vi "DraftOCU.vi"() -> ()   [LabVIEW 2013]
doc: "Inputs from the control panel to the MDF \nOutputs an object\nWhen a button is pressed, creates and MDF object (based on information typed in by hand on the control panel) and adds it to a Q\nLimitations:????\nCreators: Bocamazo and Coleman\nDate:P 11/8/2013"
uses:
  RIO-OCU_Comm/NetworkStreams/Writer/NetworkStreamWriter.lvclass
  cRIO_Code/Logic/Classes/Missions/GenericMission/GenericMission.lvclass
  RIO-OCU_Comm/ToRIO.ctl
  Location of Think.ctl
  cRIO_Code/Data/TypeDefs/UTM Location.ctl
  cRIO_Code/Data/TypeDefs/MissionTypeControl.ctl
panel:
  in  "stop":bool
  in  "Mission Type":T1
  in  "Points of Interest":T2[](array[typedef]) {"North" format="%#_10f"; "East" format="%#_8f"}
  in  "Tolerance (m)":dbl
  in  "Duration (s)":dbl=-1.0
  in  "Timeout (s)":dbl=-1.0
  in  "OK Button":bool
  in  "Error In":errorcluster
  in  "stop 2":bool
  out "Connected?":bool
  in  "Location of THINK":T3="127.0.0.1"
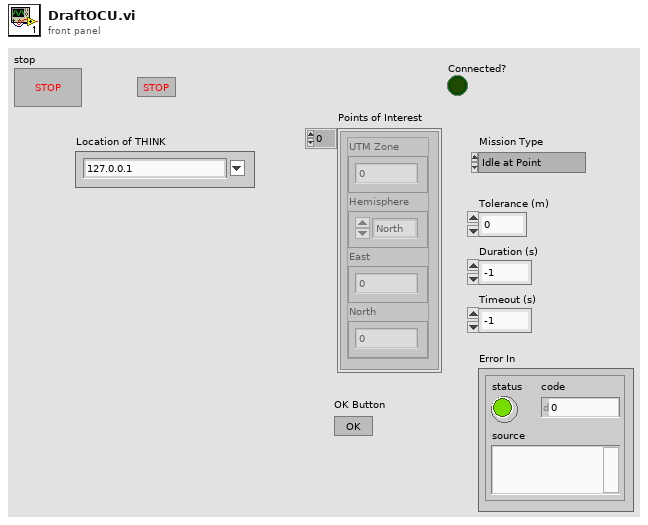
[diagram p1: front panel]
types:
  T1 = typedef "MissionTypeControl.ctl" = enum16{"Idle at Point", "Drive to Waypoint", "Round Buoy to Port", "Round Buoy to Starboard", "Pass Between Buoys", "Station Keeping"}
  T2 = typedef "UTM Location.ctl" = cluster{"UTM Zone":dbl, "Hemisphere":enum16{"North", "South"}, "East":dbl, "North":dbl}
  T3 = typedef "Location of Think.ctl" = string
  T4 = typedef "ToRIO.ctl" = cluster{"Mission":refnum<class "GenericMission.lvclass">}
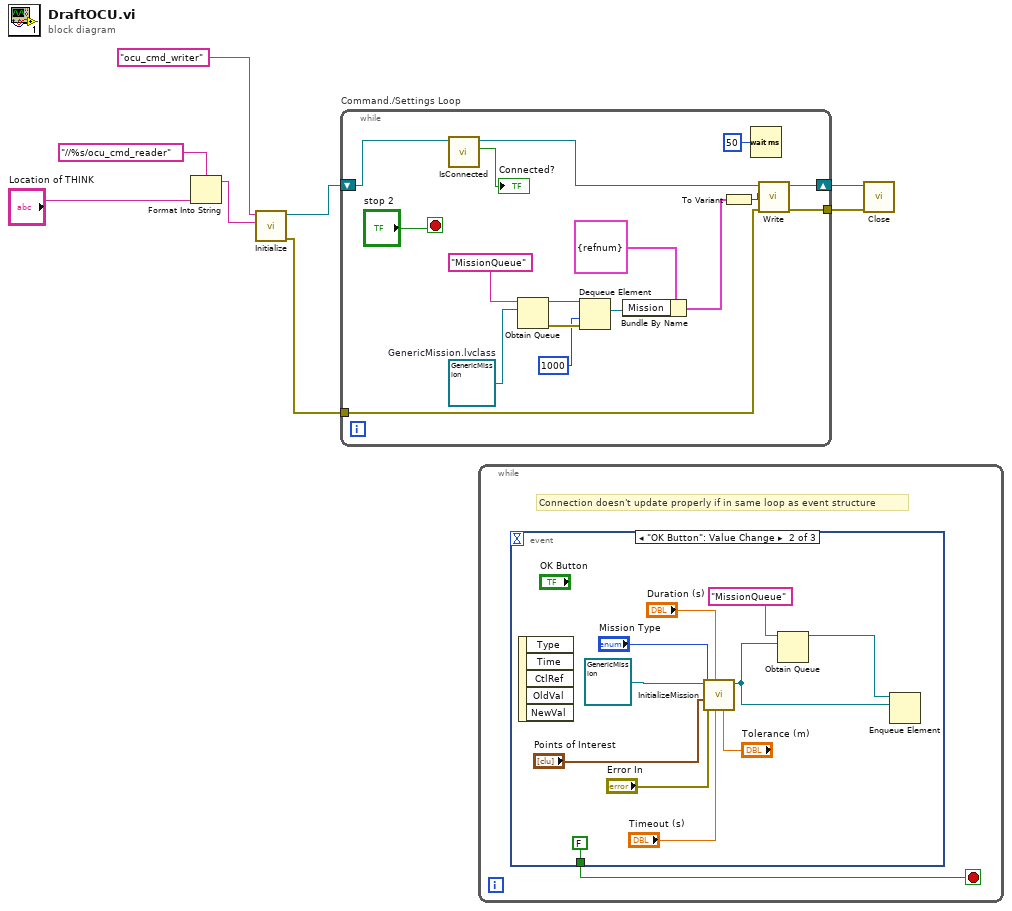
[diagram p0: block diagram]
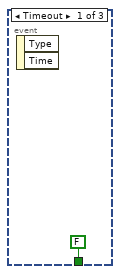
[diagram p2: hidden frame]
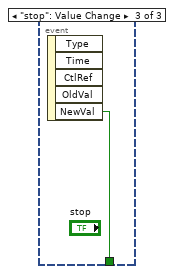
[diagram p3: hidden frame]
diagram:
  n1 = Format Into String(format string="//%s/ocu_cmd_reader", "Location of THINK") -> (resulting string=w7:string)  [unwired: 2 in, 1 out]
  n2 = call "Initialize.vi"("reader url"=w7, "writer name"="ocu_cmd_writer") -> ("error out"=w1:errorcluster, "NetworkStreamWriter out"=w2:refnum<class "NetworkStreamWriter.lvclass">)  [unwired: 8 in]
  n3 = while "Command./Settings Loop" {
    tunnel: [w16] -> w3
    shift-right: [w17] -> w4
    shift-left: w2 -> [w13]
    tunnel: w1 -> [w14]
    stop <- "stop 2" stop-if-true
    w18 = refnum<class "GenericMission.lvclass"> refnum  # GenericMission.lvclass
    n4 = call "IsConnected.vi"("NetworkStreamWriter in"=w13) -> ("Connected?"=→"Connected?":bool, "NetworkStreamWriter out"=w12:refnum<class "NetworkStreamWriter.lvclass">)  [unwired: 8 in, 1 out]
    n5 = Obtain Queue(name (unnamed)="MissionQueue", element data type=w18) -> (queue out=w24:refnum<queue>, error out=w23:errorcluster)  [unwired: 3 in, 1 out]
    n6 = Dequeue Element(queue=w24, timeout in ms (-1)=1000, error in (no error)=w23) -> (element=w22:refnum<class "GenericMission.lvclass">)  [unwired: 3 out]
    n7 = Bundle By Name(cluster=T4 {"Mission"=refnum} ("To RIO"), "Mission"=w22) -> (w19:T4)
    n8 = To Variant(anything=w19) -> (Variant=w20:variant)
    n9 = Wait (ms)(milliseconds to wait=u32 50) -> ()  [unwired: 1 out]
    n10 = call "Write.vi"("error in (no error)"=w14, "element"=w20, "NetworkStreamWriter in"=w12) -> ("error out"=w16:errorcluster, "NetworkStreamWriter out"=w17:refnum<class "NetworkStreamWriter.lvclass">)  [unwired: 7 in]
  }
  n11 = while {
    stop <- w26 stop-if-true
    # "Connection doesn't update properly if in same loop as event structure"
    n12 = event shown="[1] \"OK Button\": Value Change" {
      selector: _ -> [_ _ _]
      dyn-events: _ -> [_ _ _]
      timeout: _ -> [_ _ _]
      tunnel: [FALSE ("NewVal") FALSE ("NewVal") w39] -> w26
      event Timeout {
        n13 = event-data() -> ()  [unwired: 1 in, 2 out]
      }
      event "OK Button": Value Change {
        n14 = event-data() -> ()  [unwired: 1 in, 5 out]
        n15 = call-dynamic "InitializeMission.vi"("Tolerance (m)"="Tolerance (m)", "Timeout (s)"="Timeout (s)", "Duration (s)"="Duration (s)", "Error In"="Error In", "Points of Interest"="Points of Interest", "Mission Type"="Mission Type", "GenericMission in"=refnum<class "GenericMission.lvclass"> refnum) -> ("GenericMission out"=w37:refnum<class "GenericMission.lvclass">)  [unwired: 3 in, 1 out]
        n16 = Obtain Queue(name (unnamed)="MissionQueue", element data type=w37) -> (queue out=w38:refnum<queue>)  [unwired: 3 in, 2 out]
        n17 = Enqueue Element(queue=w38, element=w37) -> ()  [unwired: 2 in, 3 out]
      }
      event "stop": Value Change {
        n18 = event-data() -> ("NewVal"=w39:bool)  [unwired: 1 in, 4 out]
      }
    }
  }
  n19 = call "Close.vi"("error in (no error)"=w3, "NetworkStreamWriter in"=w4) -> ()  [unwired: 9 in, 1 out]
